vi "Initialize Sessions.vi"(0 "Session Handle in":T1, 5 "Baud Rate":u32=250000, 7 "Termination":u32(ring)=1 items=["Off", "On"], 9 "CAN Interface":refnum<k21>="CAN1", 11 "error in (no error)":errorcluster) -> (4 "Session Handle Out":T1, 15 "error out":errorcluster)   [LabVIEW 2015, in "PAS.lvclass"]
uses:
  PAS.lvclass
  Typedefs/Session Handle.ctl
  PAS.lvclass/PAS.ctl
  <vilib>/xnet/xnet.llb/XNET Create Session (Frame Output Stream).vi
  <vilib>/xnet/xnet.llb/XNET Create Session (Frame Input Stream).vi
  <resource>/objmgr/xnet.rc
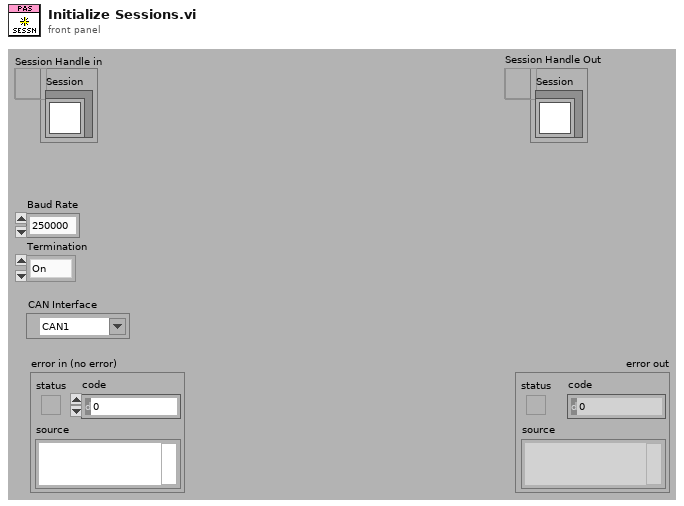
[diagram p1: front panel]
types:
  T1 = typedef "PAS.lvclass/Session Handle.ctl" = refnum<data-value>
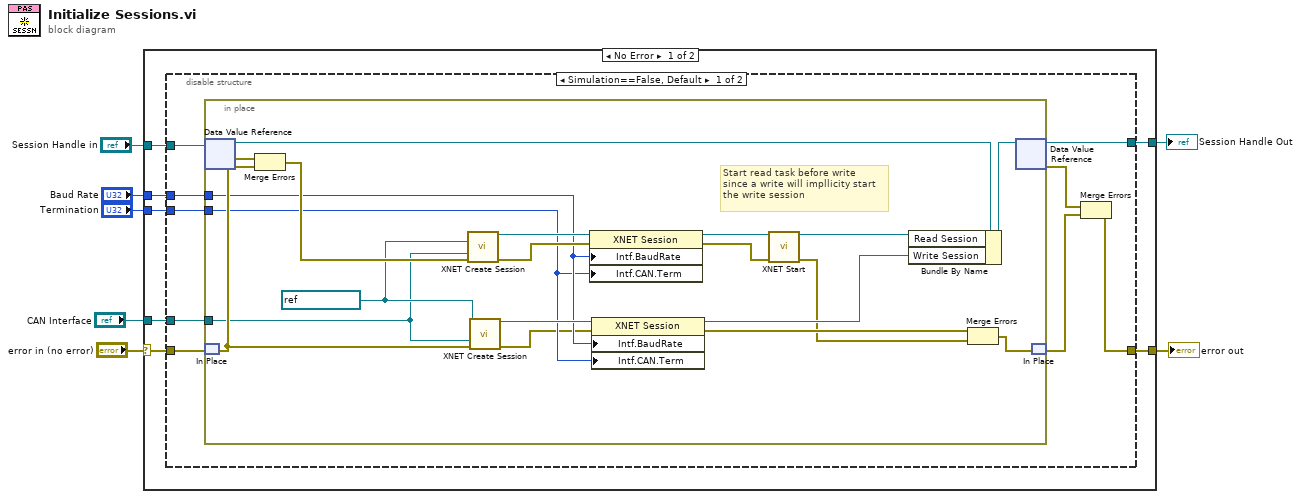
[diagram p0: block diagram]
diagram:
  n1 = case shown="No Error" "error in (no error)" {
    selector: "error in (no error)" -> [w13 w47]
    tunnel: [w14 w47] -> w7
    tunnel: "Baud Rate" -> [w12 _]
    tunnel: "Termination" -> [w11 _]
    tunnel: "Session Handle in" -> [w10 w46]
    tunnel: [w9 w46] -> w2
    tunnel: "CAN Interface" -> [w8 _]
    frame No Error {
      n2 = disable-structure shown="Simulation==False, Default" {
        disable-tunnel: [w21 w44] -> w14
        disable-tunnel: w13 -> [w20 w44]
        disable-tunnel: w12 -> [w19 _]
        disable-tunnel: w11 -> [w18 _]
        disable-tunnel: w10 -> [w17 w45]
        disable-tunnel: [w16 w45] -> w9
        disable-tunnel: w8 -> [w15 _]
        frame condition #0 (active) {
          n3 = in-place {
            in-place-border: w19 -> [w36]
            in-place-border: w18 -> [w35]
            in-place-border: w15 -> [w24]
            w41 = refnum<k21> ":memory:" ("CAN Cluster")
            # "Start read task before write\nsince a write will impllicity start\nthe write session"
            n4 = in-place-dvr #1(w17) -> (w26:refnum<class "PAS.lvclass">, w43:errorcluster)
            n5 = in-place-match #2(w20) -> (w40:errorcluster)
            n6 = Merge Errors(w40, w43) -> (w42:errorcluster)
            n7 = call-poly <vilib>:"XNET Create Session.vi"("cluster (:memory:)"=w41, "interface"=w24, "error in (no error)"=w42) -> ("session out"=w39:refnum<k21>, "error out"=w38:errorcluster)  [unwired: 11 out]
            n8 = call-poly <vilib>:"XNET Create Session.vi"("cluster (:memory:)"=w41, "interface"=w24, "error in (no error)"=w40) -> ("session out"=w37:refnum<k21>, "error out"=w34:errorcluster)  [unwired: 11 out]
            n9 = property class="XNET Session"(reference=w39, error in=w38, "Intf.BaudRate"=w36, "Intf.CAN.Term"=w35) -> (reference out=w30:refnum<k21>, error out=w29:errorcluster)
            n10 = property class="XNET Session"(reference=w37, error in=w34, "Intf.BaudRate"=w36, "Intf.CAN.Term"=w35) -> (reference out=w33:refnum<k21>, error out=w32:errorcluster)
            n11 = call <vilib>:"XNET Start.vi"("session in"=w30, "error in (no error)"=w29) -> ("session out"=w28:refnum<k21>, "error out"=w27:errorcluster)  [unwired: 12 in]
            n12 = Bundle By Name(cluster=w26, "Read Session"=w28, "Write Session"=w33) -> (w25:refnum<class "PAS.lvclass">)
            n13 = Merge Errors(w32, w27) -> (w31:errorcluster)
            n14 = in-place-dvr #1(w25) -> (w16:T1, w22:errorcluster)
            n15 = in-place-match #2(w31) -> (w23:errorcluster)
          }
          n16 = Merge Errors(w22, w23) -> (w21:errorcluster)
        }
        frame condition #1 {
        }
      }
    }
    frame Error {
    }
  }
  "error out" <- w7
  "Session Handle Out" <- w2
